vi "DataASCFileInfo.vi"(9 "Language":u32, 11 "file path (dialog if empty)":path caption="文件路径 （空时为对话框）") -> (0 "路径输出":path, 1 "FileInfo":string, 2 "文件类型":string)   [LabVIEW 2015]
uses:
  <vilib>/regexp/Match Regular Expression.xnode
panel:
  out "总帧数 2":i32
  out "倒数第二行":string
  out "判断":string
  out "倒数第一行":string
  out "数据首行":string
  out "总帧数":i32
  out "第2行":string
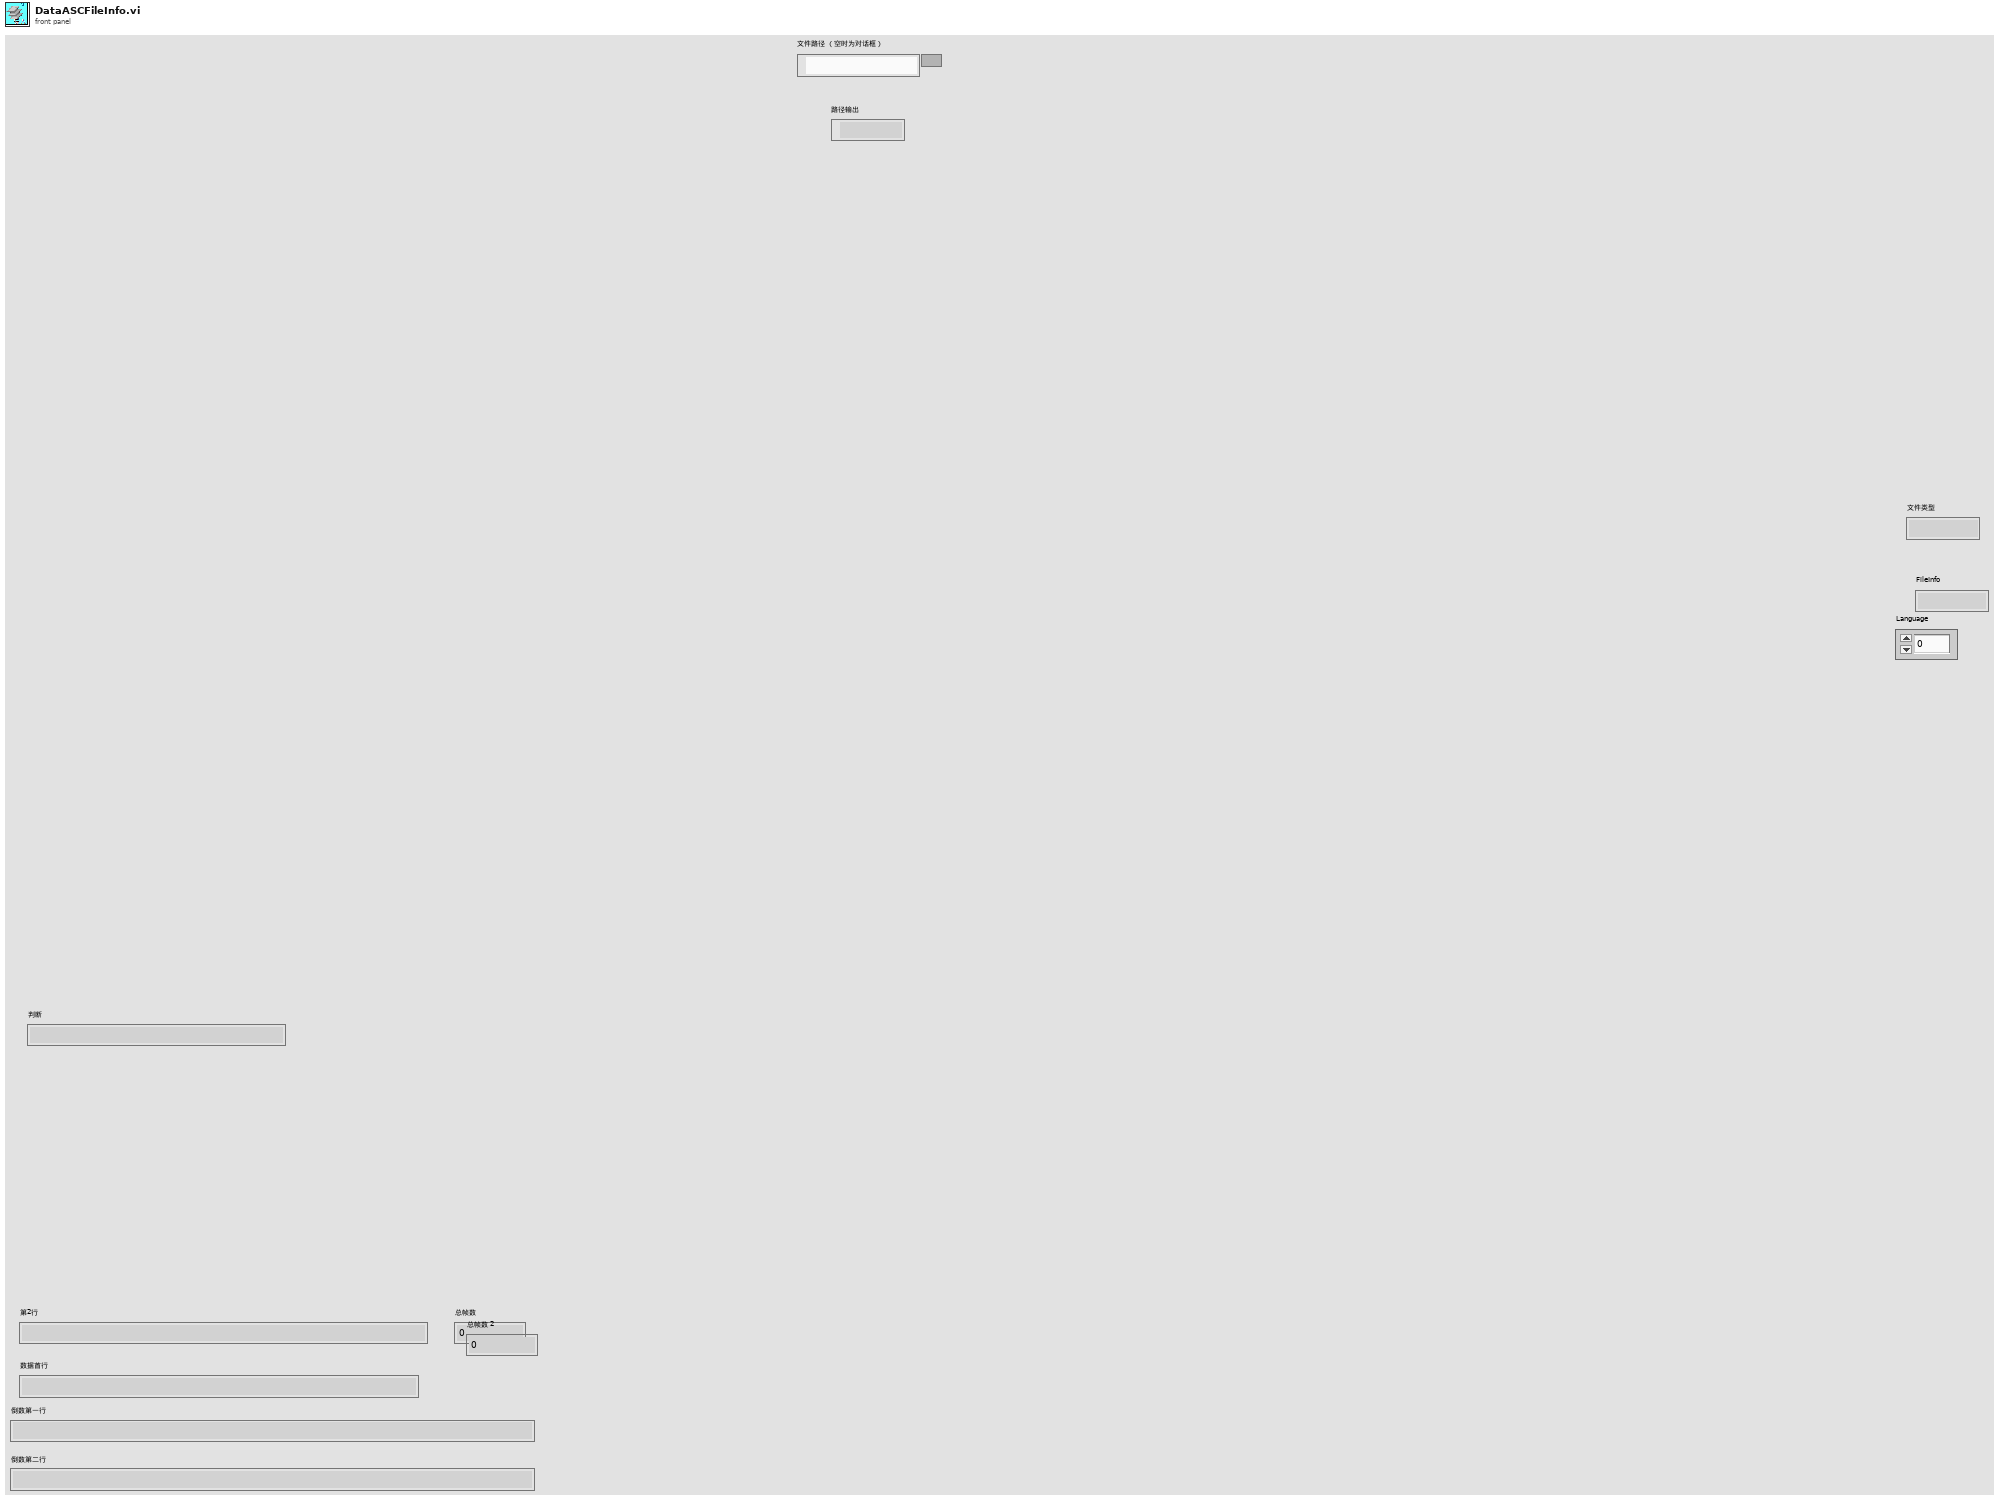
[diagram p1: front panel]
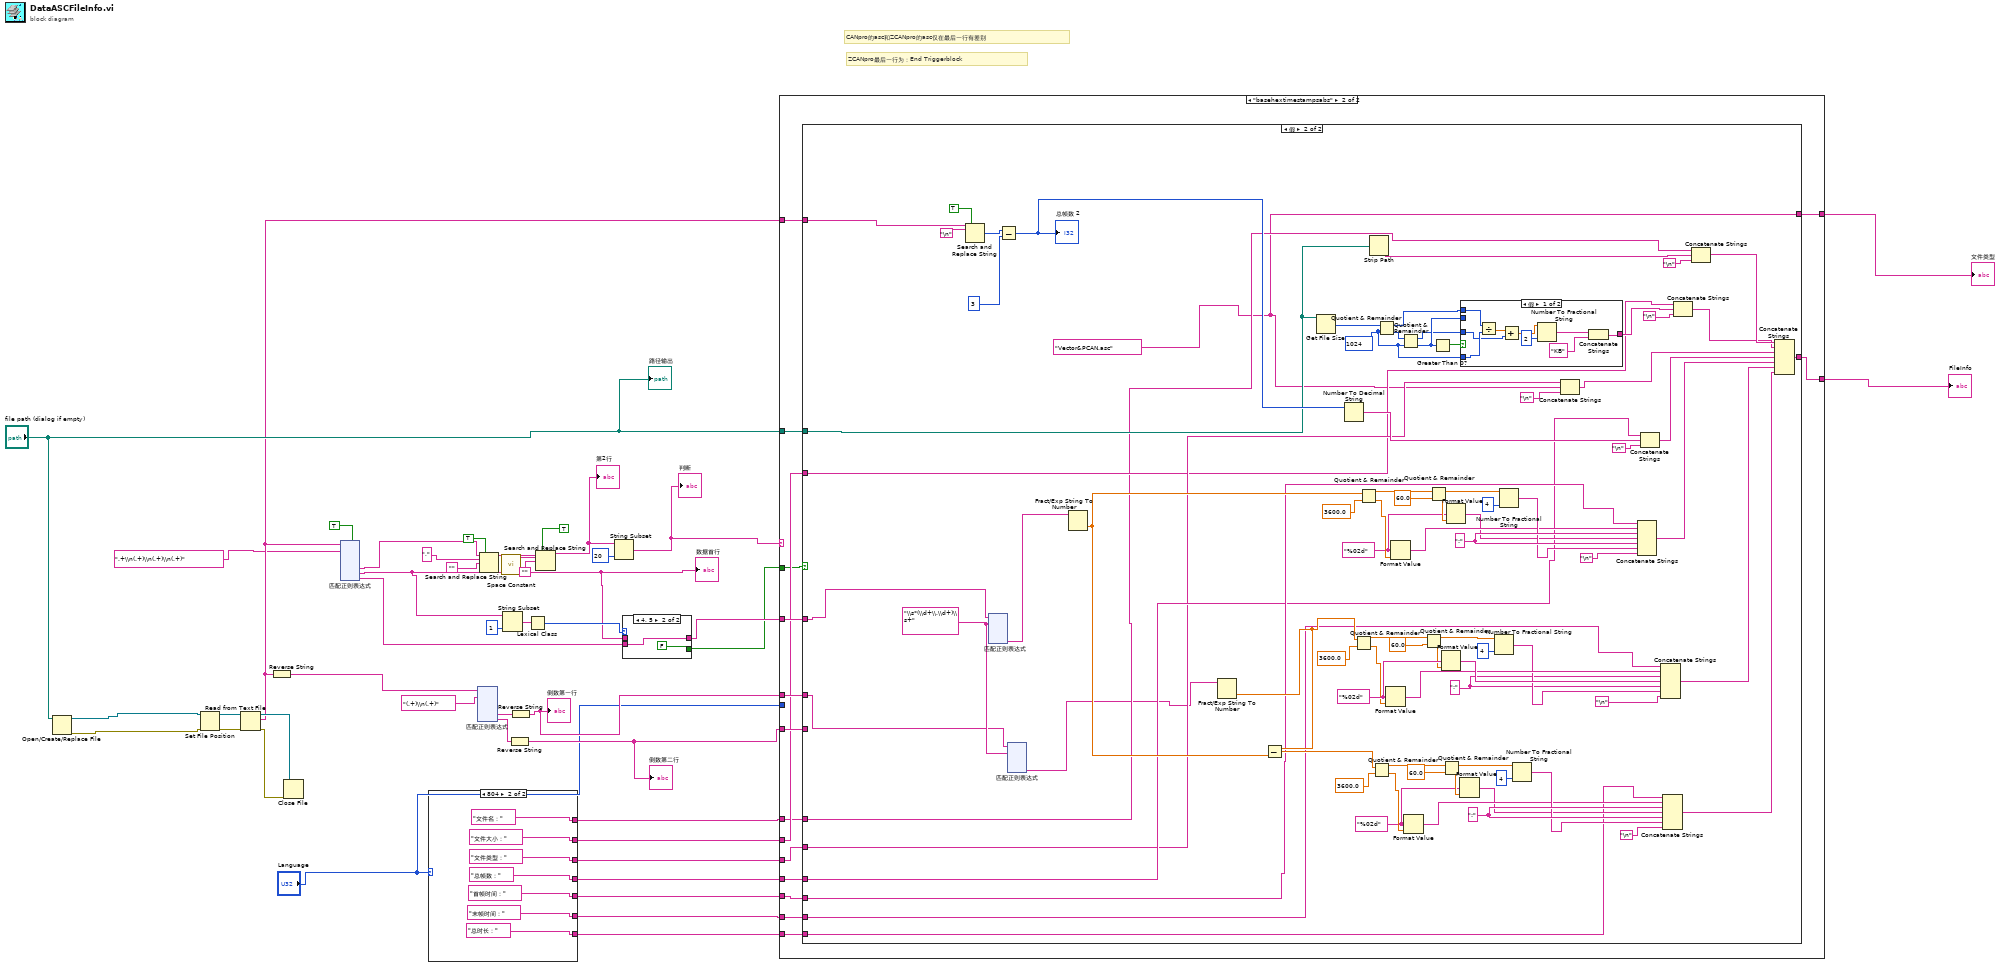
[diagram p0: block diagram]
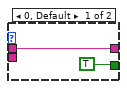
[diagram p2: hidden frame]
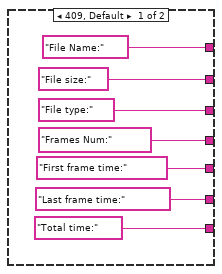
[diagram p3: hidden frame]
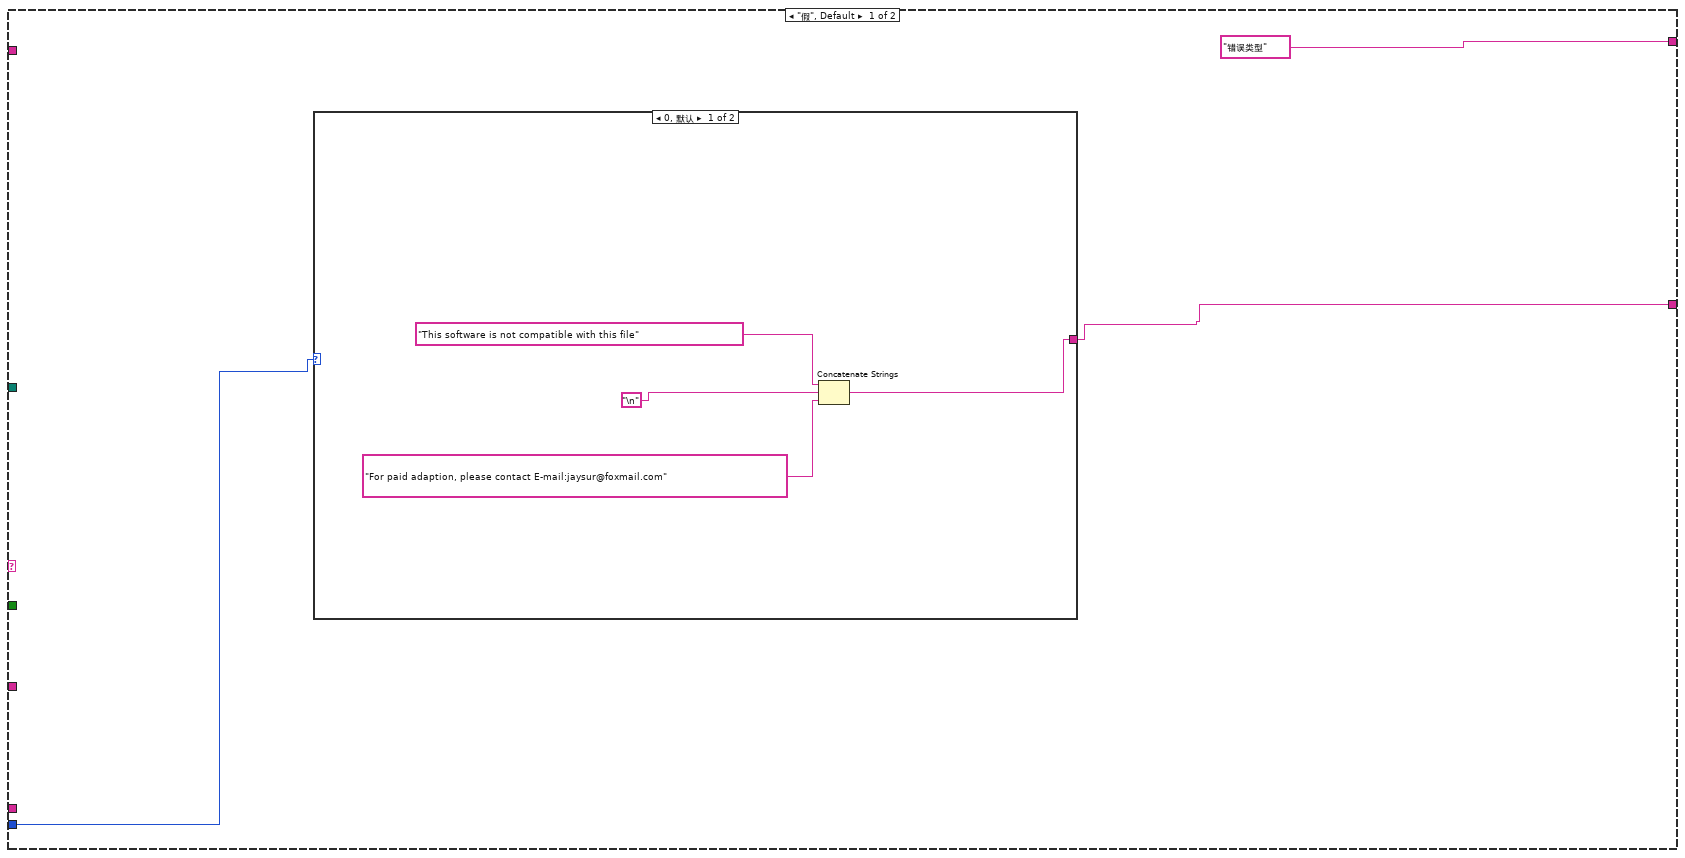
[diagram p4: hidden frame]
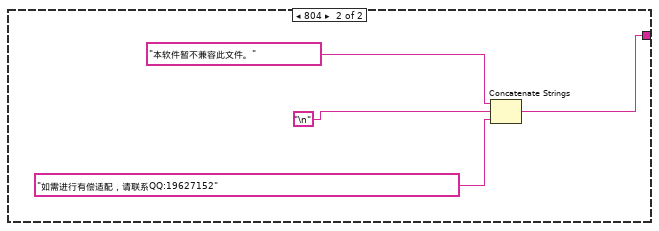
[diagram p5: hidden frame]
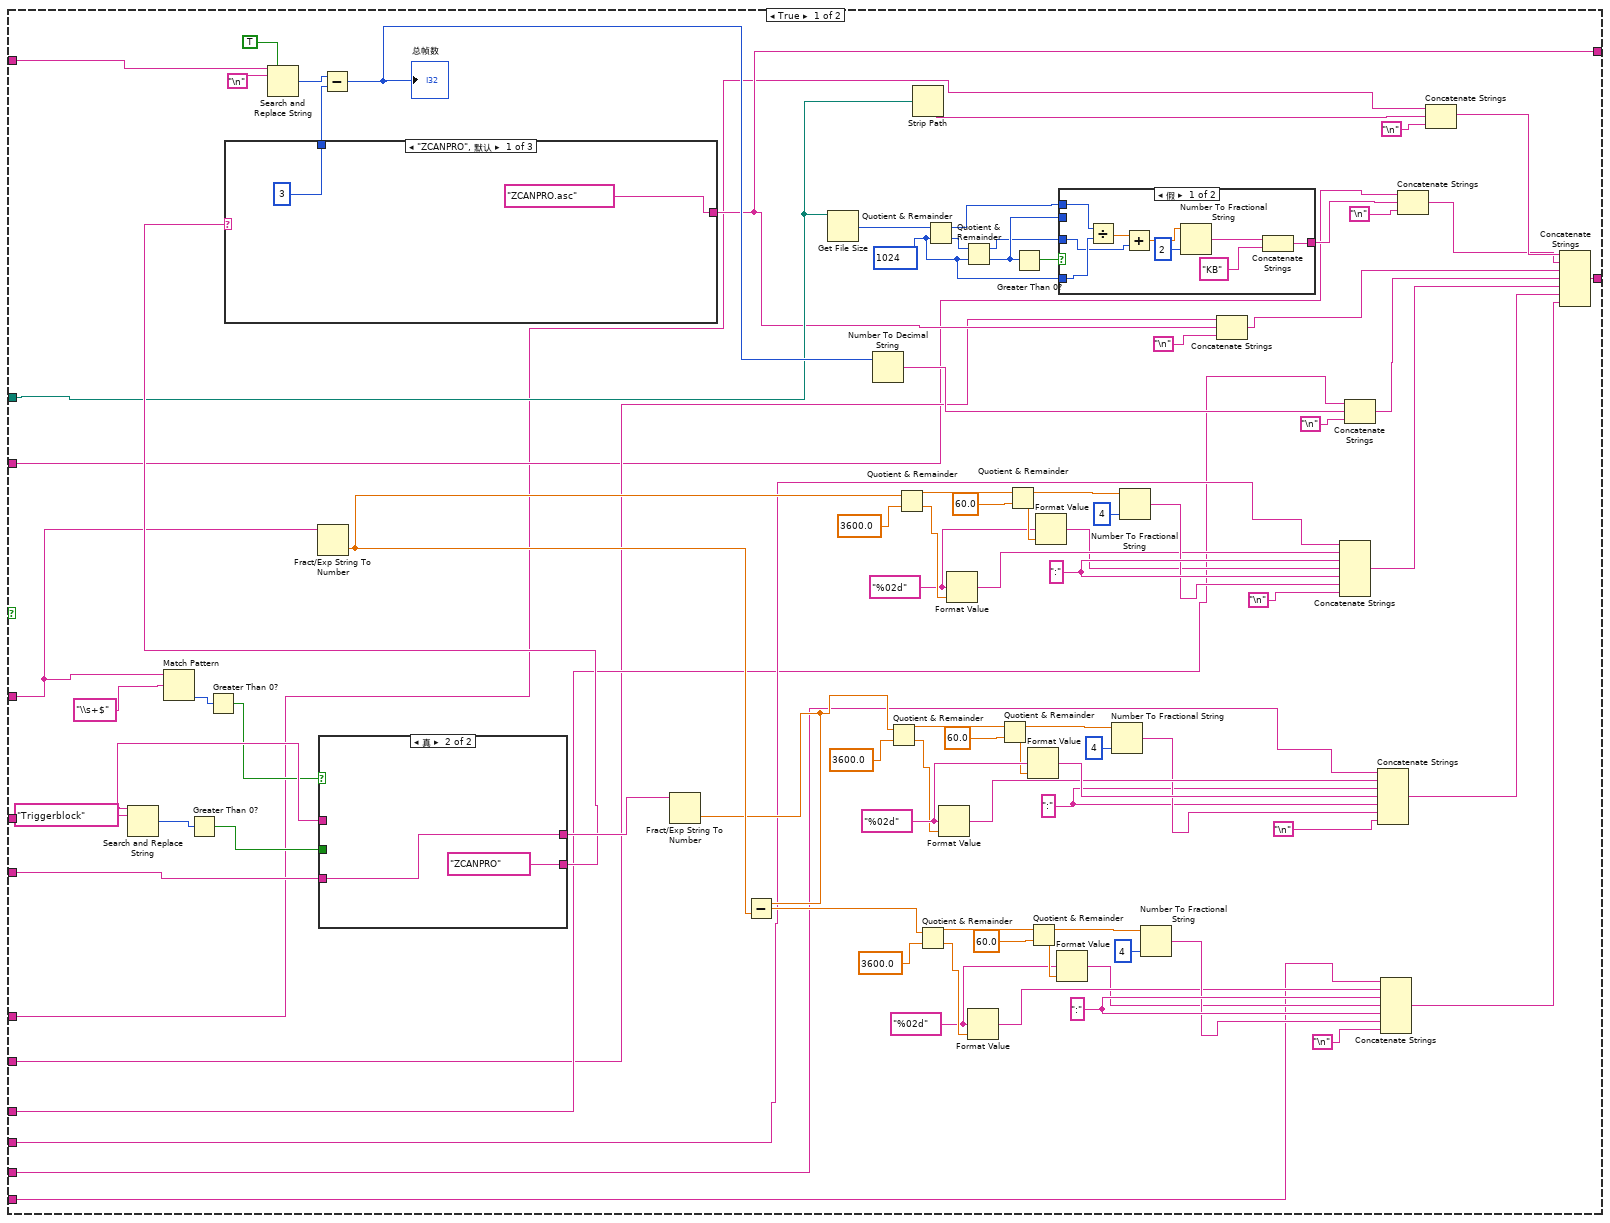
[diagram p6: hidden frame]
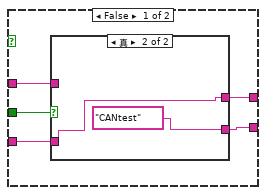
[diagram p7: hidden frame]
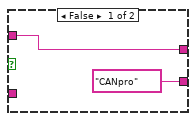
[diagram p8: hidden frame]
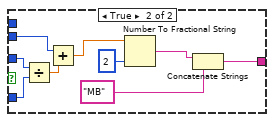
[diagram p9: hidden frame]
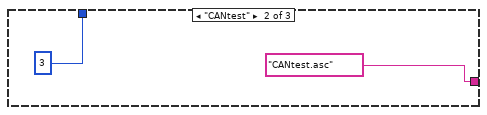
[diagram p10: hidden frame]
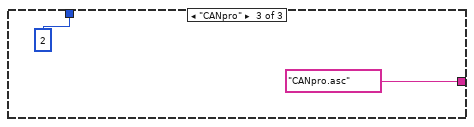
[diagram p11: hidden frame]
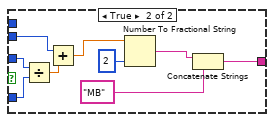
[diagram p12: hidden frame]
diagram:
  # "ZCANpro最后一行为：End Triggerblock"
  # "CANpro的asc和ZCANpro的asc仅在最后一行有差别"
  n1 = Open/Create/Replace File(file path (use dialog)="file path (dialog if empty)") -> (refnum out=w23:refnum<file>, error out=w22:errorcluster)  [unwired: 5 in, 1 out]
  n2 = Set File Position(refnum=w23, error in=w22) -> (refnum out=w42:refnum<file>, error out=w41:errorcluster)  [unwired: 2 in]
  n3 = Read from Text File(file (use dialog)=w42, error in=w41) -> (refnum out=w27:refnum<file>, text=w17:string, error out=w26:errorcluster)  [unwired: 2 in, 1 out]
  n4 = Reverse String(1:w17) -> (0:w31:string)
  n5 = Close File(refnum=w27, error in=w26) -> ()  [unwired: 2 out]
  n6 = xnode "匹配正则表达式"("输入字符串"=w17, "正则表达式"=".+\\n(.+)\\n(.+)\\n(.+)", "多行？(F)"=TRUE) -> ("子匹配 1"=w38:string, "子匹配 2"=w4:string, "子匹配 3"=w3:string)  [unwired: 3 in, 5 out]
  "数据首行" <- w4
  n7 = case shown="804" "Language" {
    tunnel: ["Total time:" "总时长："] -> w10
    tunnel: ["Last frame time:" "末帧时间："] -> w11
    tunnel: ["First frame time:" "首帧时间："] -> w12
    tunnel: ["Frames Num:" "总帧数："] -> w13
    tunnel: ["File type:" "文件类型："] -> w14
    tunnel: ["File size:" "文件大小："] -> w15
    tunnel: ["File Name:" "文件名："] -> w16
    frame 409, Default {
    }
    frame 804 {
    }
  }
  n8 = xnode "匹配正则表达式"("输入字符串"=w31, "正则表达式"="(.+)\\n(.+)") -> ("子匹配 1"=w30:string, "子匹配 2"=w24:string)  [unwired: 4 in, 5 out]
  n9 = Search and Replace String(replace all?=TRUE ("替换全部？(F)"), input string=w38, search string=",", replace string="") -> (result string=w36:string)  [unwired: 4 in, 3 out]
  n10 = call <vilib>:"Space Constant.vi"() -> ("String"=w35:string)
  n11 = String Subset(string=w4, length (rest)=1 ("长度（剩余）")) -> (substring=w7:string)  [unwired: 1 in]
  n12 = Reverse String(1:w24) -> (0:w19:string)
  "倒数第二行" <- w19
  n13 = Reverse String(1:w30) -> (0:w20:string)
  "倒数第一行" <- w20
  n14 = Lexical Class(1:w7) -> (0:w6:i16)
  n15 = Search and Replace String(replace all?=TRUE ("替换全部？(F)"), input string=w36, search string=w35, replace string="") -> (result string=w29:string)  [unwired: 4 in, 3 out]
  "第2行" <- w29
  n16 = String Subset(string=w29, length (rest)=20 ("长度（剩余）")) -> (substring=w21:string)  [unwired: 1 in]
  "判断" <- w21
  n17 = case shown="4, 5" w6 {
    tunnel: [TRUE FALSE] -> w1
    tunnel: w4 -> [w59 _]
    tunnel: [w59 w61] -> w5
    tunnel: w3 -> [_ w61]
    frame 0, Default {
    }
    frame 4, 5 {
    }
  }
  n18 = case shown="\"basehextimestampsabs\"" w21 {
    tunnel: ["错误类型" w78] -> w44
    tunnel: [w64 w88] -> w43
    tunnel: "file path (dialog if empty)" -> [_ w84]
    tunnel: w5 -> [_ w83]
    tunnel: w20 -> [_ w87]
    tunnel: w19 -> [_ w86]
    tunnel: w17 -> [_ w85]
    tunnel: w16 -> [_ w75]
    tunnel: w15 -> [_ w76]
    tunnel: w14 -> [_ w77]
    tunnel: w13 -> [_ w79]
    tunnel: w12 -> [_ w80]
    tunnel: w11 -> [_ w81]
    tunnel: w10 -> [_ w82]
    tunnel: "Language" -> [w63 _]
    tunnel: w1 -> [_ w74]
    frame "假", Default {
      n19 = case shown="0, 默认" w63 {
        tunnel: [w66 w70] -> w64
        frame 0, Default {
          n20 = Concatenate Strings("This software is not compatible with this file", "\n", "For paid adaption, please contact E-mail:jaysur@foxmail.com") -> (w66:string)
        }
        frame 804 {
          n21 = Concatenate Strings("本软件暂不兼容此文件。", "\n", "如需进行有偿适配，请联系QQ:19627152") -> (w70:string)
        }
      }
    }
    frame "basehextimestampsabs" {
      n22 = case shown="假" w74 {
        tunnel: [w166 w285] -> w88
        tunnel: w87 -> [w113 w216]
        tunnel: w86 -> [w110 _]
        tunnel: w85 -> [w105 w230]
        tunnel: w84 -> [w102 w227]
        tunnel: w83 -> [w100 w214]
        tunnel: w82 -> [w96 w226]
        tunnel: w81 -> [w95 w225]
        tunnel: w80 -> [w94 w224]
        tunnel: w79 -> [w93 w223]
        tunnel: [w92 w219] -> w78
        tunnel: w77 -> [w91 w222]
        tunnel: w76 -> [w90 w221]
        tunnel: w75 -> [w89 w220]
        frame True {
          w121 = i64 1024 ("y")
          w140 = "%02d" ("格式字符串")
          w146 = ":"
          w164 = "%02d" ("格式字符串")
          w158 = ":"
          w167 = "%02d" ("格式字符串")
          w173 = ":"
          n23 = Search and Replace String(input string=w113, search string="Triggerblock" ("搜索字符串")) -> (number of replacements=w115:i32)  [unwired: 6 in, 3 out]
          n24 = Match Pattern(string=w100, regular expression="\\s+$") -> (offset past match=w99:i32)  [unwired: 1 in, 3 out]
          n25 = Greater Than 0?(x=w115) -> (x > 0?=w97:bool)
          n26 = Greater Than 0?(x=w99) -> (x > 0?=w98:bool)
          n27 = Search and Replace String(replace all?=TRUE ("替换全部？(F)"), input string=w105, search string="\n") -> (number of replacements=w107:i32)  [unwired: 5 in, 3 out]
          n28 = Fract/Exp String To Number(string=w100) -> (number=w116:dbl)  [unwired: 3 in, 1 out]
          n29 = case shown="真" w98 {
            tunnel: [w182 w189] -> w112
            tunnel: w110 -> [w179 w189]
            tunnel: [w183 "ZCANPRO"] -> w109
            tunnel: w113 -> [w181 _]
            tunnel: w97 -> [w180 _]
            frame False {
              n30 = case shown="真" w180 {
                tunnel: ["CANpro" "CANtest"] -> w183
                tunnel: [w184 w187] -> w182
                tunnel: w181 -> [w184 _]
                tunnel: w179 -> [_ w187]
                frame False {
                }
                frame True {
                }
              }
            }
            frame True {
            }
          }
          n31 = case shown="\"ZCANPRO\", 默认" w109 {
            tunnel: ["ZCANPRO.asc" "CANtest.asc" "CANpro.asc"] -> w92
            tunnel: [3 ("y") 3 ("y") 2 ("y")] -> w104
            frame "ZCANPRO", Default {
            }
            frame "CANtest" {
            }
            frame "CANpro" {
            }
          }
          n32 = Subtract(x=w107, y=w104) -> (x-y=w103:i32)
          "总帧数" <- w103
          n33 = Fract/Exp String To Number(string=w112) -> (number=w111:dbl)  [unwired: 3 in, 1 out]
          n34 = Subtract(x=w111, y=w116) -> (x-y=w139:dbl)
          n35 = Get File Size(file=w102) -> (size (in bytes)=w124:i64)  [unwired: 1 in, 2 out]
          n36 = Number To Decimal String(number=w103) -> (decimal integer string=w127:string)  [unwired: 1 in]
          n37 = Quotient & Remainder(x=w111, y=3600.0) -> (x-y*floor(x/y)=w154:dbl, floor(x/y)=w161:dbl)
          n38 = Quotient & Remainder(x=w116, y=3600.0) -> (x-y*floor(x/y)=w177:dbl, floor(x/y)=w170:dbl)
          n39 = Strip Path(path=w102) -> (name=w134:string)  [unwired: 1 out]
          n40 = Quotient & Remainder(x=w139, y=3600.0) -> (x-y*floor(x/y)=w150:dbl, floor(x/y)=w143:dbl)
          n41 = Quotient & Remainder(x=w124, y=w121) -> (x-y*floor(x/y)=w117:i64, floor(x/y)=w123:i64)
          n42 = Format Value(format string=w164, value (0)=w161) -> (output string=w160:string)  [unwired: 1 in]
          n43 = Format Value(format string=w167, value (0)=w170) -> (output string=w171:string)  [unwired: 1 in]
          n44 = Quotient & Remainder(x=w123, y=w121) -> (x-y*floor(x/y)=w119:i64, floor(x/y)=w120:i64)
          n45 = Format Value(format string=w140, value (0)=w143) -> (output string=w144:string)  [unwired: 1 in]
          n46 = Quotient & Remainder(x=w154, y=60.0) -> (x-y*floor(x/y)=w156:dbl, floor(x/y)=w162:dbl)
          n47 = Quotient & Remainder(x=w177, y=60.0) -> (x-y*floor(x/y)=w175:dbl, floor(x/y)=w169:dbl)
          n48 = Greater Than 0?(x=w120) -> (x > 0?=w122:bool)
          n49 = Format Value(format string=w164, value (0)=w162) -> (output string=w163:string)  [unwired: 1 in]
          n50 = Quotient & Remainder(x=w150, y=60.0) -> (x-y*floor(x/y)=w148:dbl, floor(x/y)=w142:dbl)
          n51 = Format Value(format string=w167, value (0)=w169) -> (output string=w168:string)  [unwired: 1 in]
          n52 = Format Value(format string=w140, value (0)=w142) -> (output string=w141:string)  [unwired: 1 in]
          n53 = case shown="假" w122 {
            tunnel: w121 -> [w195 w205]
            tunnel: w120 -> [_ w203]
            tunnel: w119 -> [w193 w206]
            tunnel: [w198 w201] -> w118
            tunnel: w117 -> [w196 _]
            frame False {
              n54 = Divide(x=w196, y=w195) -> (x/y=w194:dbl)
              n55 = Add(x=w194, y=w193) -> (x+y=w192:dbl)
              n56 = Number To Fractional String(number=w192, precision (6)=i16 2 ("精度(6)")) -> (F-format string=w190:string)  [unwired: 2 in]
              n57 = Concatenate Strings(w190, "KB" ("字符串")) -> (w198:string)
            }
            frame True {
              n58 = Divide(x=w206, y=w205) -> (x/y=w204:dbl)
              n59 = Add(x=w203, y=w204) -> (x+y=w202:dbl)
              n60 = Number To Fractional String(number=w202, precision (6)=i16 2 ("精度(6)")) -> (F-format string=w200:string)  [unwired: 2 in]
              n61 = Concatenate Strings(w200, "MB") -> (w201:string)
            }
          }
          n62 = Number To Fractional String(number=w156, precision (6)=i16 4 ("精度(6)")) -> (F-format string=w159:string)  [unwired: 2 in]
          n63 = Number To Fractional String(number=w175, precision (6)=i16 4 ("精度(6)")) -> (F-format string=w172:string)  [unwired: 2 in]
          n64 = Number To Fractional String(number=w148, precision (6)=i16 4 ("精度(6)")) -> (F-format string=w145:string)  [unwired: 2 in]
          n65 = Concatenate Strings(w91, w92, "\n") -> (w131:string)
          n66 = Concatenate Strings(w94, w171, w173, w168, w173, w172, "\n") -> (w165:string)
          n67 = Concatenate Strings(w93, w127, "\n") -> (w128:string)
          n68 = Concatenate Strings(w95, w160, w158, w163, w158, w159, "\n") -> (w152:string)
          n69 = Concatenate Strings(w96, w144, w146, w141, w146, w145, "\n") -> (w138:string)
          n70 = Concatenate Strings(w90, w118, "\n") -> (w125:string)
          n71 = Concatenate Strings(w89, w134, "\n") -> (w133:string)
          n72 = Concatenate Strings(w133, w125, w131, w128, w165, w152, w138) -> (w166:string)
        }
        frame False {
          w218 = "\\s*(\\d+\\.\\d+)\\s+" ("正则表达式")
          w219 = "Vector&PCAN.asc"
          w240 = i64 1024 ("y")
          w259 = "%02d" ("格式字符串")
          w265 = ":"
          w283 = "%02d" ("格式字符串")
          w277 = ":"
          w286 = "%02d" ("格式字符串")
          w292 = ":"
          n73 = Search and Replace String(replace all?=TRUE ("替换全部？(F)"), input string=w230, search string="\n") -> (number of replacements=w232:i32)  [unwired: 5 in, 3 out]
          n74 = xnode "匹配正则表达式"("输入字符串"=w214, "正则表达式"=w218) -> ("子匹配 1"=w217:string)  [unwired: 4 in, 5 out]
          n75 = Subtract(x=w232, y=3) -> (x-y=w228:i32)
          "总帧数 2" <- w228
          n76 = xnode "匹配正则表达式"("输入字符串"=w216, "正则表达式"=w218) -> ("子匹配 1"=w215:string)  [unwired: 4 in, 5 out]
          n77 = Fract/Exp String To Number(string=w217) -> (number=w235:dbl)  [unwired: 3 in, 1 out]
          n78 = Fract/Exp String To Number(string=w215) -> (number=w234:dbl)  [unwired: 3 in, 1 out]
          n79 = Subtract(x=w234, y=w235) -> (x-y=w258:dbl)
          n80 = Get File Size(file=w227) -> (size (in bytes)=w243:i64)  [unwired: 1 in, 2 out]
          n81 = Number To Decimal String(number=w228) -> (decimal integer string=w246:string)  [unwired: 1 in]
          n82 = Quotient & Remainder(x=w234, y=3600.0) -> (x-y*floor(x/y)=w273:dbl, floor(x/y)=w280:dbl)
          n83 = Quotient & Remainder(x=w235, y=3600.0) -> (x-y*floor(x/y)=w296:dbl, floor(x/y)=w289:dbl)
          n84 = Strip Path(path=w227) -> (name=w253:string)  [unwired: 1 out]
          n85 = Quotient & Remainder(x=w258, y=3600.0) -> (x-y*floor(x/y)=w269:dbl, floor(x/y)=w262:dbl)
          n86 = Quotient & Remainder(x=w243, y=w240) -> (x-y*floor(x/y)=w236:i64, floor(x/y)=w242:i64)
          n87 = Format Value(format string=w283, value (0)=w280) -> (output string=w279:string)  [unwired: 1 in]
          n88 = Format Value(format string=w286, value (0)=w289) -> (output string=w290:string)  [unwired: 1 in]
          n89 = Quotient & Remainder(x=w242, y=w240) -> (x-y*floor(x/y)=w238:i64, floor(x/y)=w239:i64)
          n90 = Format Value(format string=w259, value (0)=w262) -> (output string=w263:string)  [unwired: 1 in]
          n91 = Quotient & Remainder(x=w273, y=60.0) -> (x-y*floor(x/y)=w275:dbl, floor(x/y)=w281:dbl)
          n92 = Quotient & Remainder(x=w296, y=60.0) -> (x-y*floor(x/y)=w294:dbl, floor(x/y)=w288:dbl)
          n93 = Greater Than 0?(x=w239) -> (x > 0?=w241:bool)
          n94 = Format Value(format string=w283, value (0)=w281) -> (output string=w282:string)  [unwired: 1 in]
          n95 = Quotient & Remainder(x=w269, y=60.0) -> (x-y*floor(x/y)=w267:dbl, floor(x/y)=w261:dbl)
          n96 = Format Value(format string=w286, value (0)=w288) -> (output string=w287:string)  [unwired: 1 in]
          n97 = Format Value(format string=w259, value (0)=w261) -> (output string=w260:string)  [unwired: 1 in]
          n98 = case shown="假" w241 {
            tunnel: w240 -> [w535 w545]
            tunnel: w239 -> [_ w543]
            tunnel: w238 -> [w533 w546]
            tunnel: [w538 w541] -> w237
            tunnel: w236 -> [w536 _]
            frame False {
              n99 = Divide(x=w536, y=w535) -> (x/y=w534:dbl)
              n100 = Add(x=w534, y=w533) -> (x+y=w532:dbl)
              n101 = Number To Fractional String(number=w532, precision (6)=i16 2 ("精度(6)")) -> (F-format string=w530:string)  [unwired: 2 in]
              n102 = Concatenate Strings(w530, "KB" ("字符串")) -> (w538:string)
            }
            frame True {
              n103 = Divide(x=w546, y=w545) -> (x/y=w544:dbl)
              n104 = Add(x=w543, y=w544) -> (x+y=w542:dbl)
              n105 = Number To Fractional String(number=w542, precision (6)=i16 2 ("精度(6)")) -> (F-format string=w540:string)  [unwired: 2 in]
              n106 = Concatenate Strings(w540, "MB") -> (w541:string)
            }
          }
          n107 = Number To Fractional String(number=w275, precision (6)=i16 4 ("精度(6)")) -> (F-format string=w278:string)  [unwired: 2 in]
          n108 = Number To Fractional String(number=w294, precision (6)=i16 4 ("精度(6)")) -> (F-format string=w291:string)  [unwired: 2 in]
          n109 = Number To Fractional String(number=w267, precision (6)=i16 4 ("精度(6)")) -> (F-format string=w264:string)  [unwired: 2 in]
          n110 = Concatenate Strings(w222, w219, "\n") -> (w250:string)
          n111 = Concatenate Strings(w224, w290, w292, w287, w292, w291, "\n") -> (w284:string)
          n112 = Concatenate Strings(w223, w246, "\n") -> (w247:string)
          n113 = Concatenate Strings(w225, w279, w277, w282, w277, w278, "\n") -> (w271:string)
          n114 = Concatenate Strings(w226, w263, w265, w260, w265, w264, "\n") -> (w257:string)
          n115 = Concatenate Strings(w221, w237, "\n") -> (w244:string)
          n116 = Concatenate Strings(w220, w253, "\n") -> (w252:string)
          n117 = Concatenate Strings(w252, w244, w250, w247, w284, w271, w257) -> (w285:string)
        }
      }
    }
  }
  "FileInfo" <- w43
  "文件类型" <- w44
  "路径输出" <- "file path (dialog if empty)"
